vi "Oscilloscope_Info_Guide.vi"() -> ()   [LabVIEW 2020]
uses:
  Return_To_Interface.ctl
panel:
  in  "Return to Interface":T1
  # "Play: Run the oscilloscope if it was stopped.\n\nPause: Pause the execution of the programme.\n\nStop: End the programme when pressed.\n\nSave: Save the waveforms and memorize numeric data into a file text.\n\nSettings: Open a page when you can change the oscilloscope settings\n\nGuide: Open this page, when you can find the meaning of the buttons.\n\nChannels Activation: Four buttons that you can press in order to enable the oscilloscope channels.\n\nReturn to Interface: When pressed, lead the user to the Oscilloscope Interface\n\nSelect a Channel for the Operation: Allows you to select the channel on which to calculate the specified function.\n\nOperating Modes: Allows you to select and set the mode of operation of the instrument.\n\nChannels Synchronization: this function updates the status of the channel indicators based on the actual oscilloscope configuration."
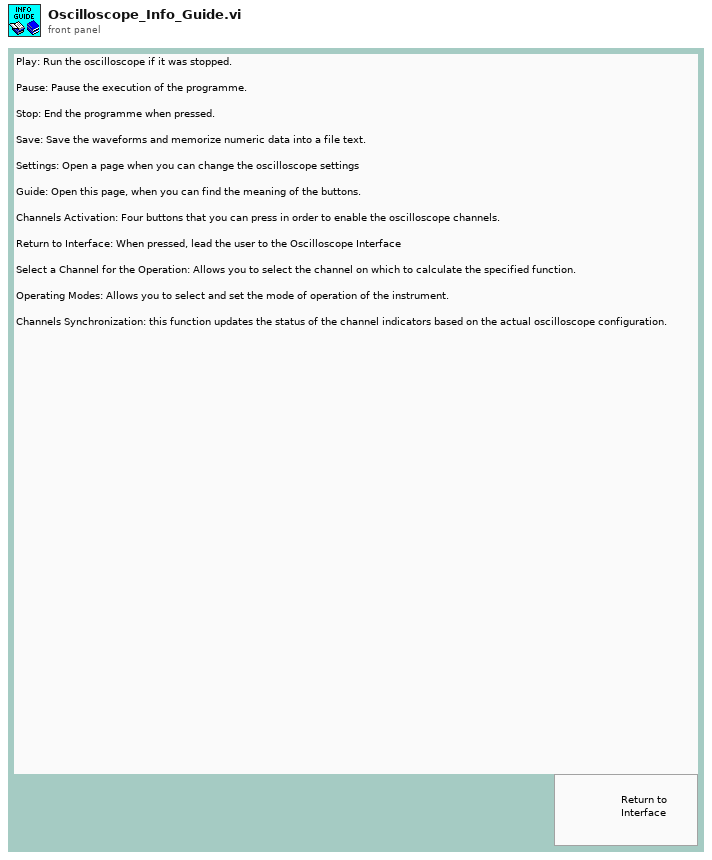
[diagram p1: front panel]
types:
  T1 = typedef "Return_To_Interface.ctl" = bool
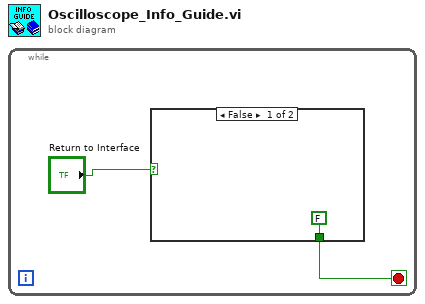
[diagram p0: block diagram]
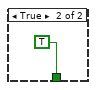
[diagram p2: hidden frame]
diagram:
  n1 = while {
    stop <- w2 stop-if-true
    n2 = case shown="False" "Return to Interface" {
      tunnel: [FALSE TRUE] -> w2
      frame False {
      }
      frame True {
      }
    }
  }
